vi "U8ToI32.vi"(4 "Index":u32, 7 "Input U8 Array":u8[](array[numeric])) -> (0 "Index+4":u32, 1 "Output I32":i32, 3 "Output U8 Array":u8[](array[numeric]))   [LabVIEW 2017]
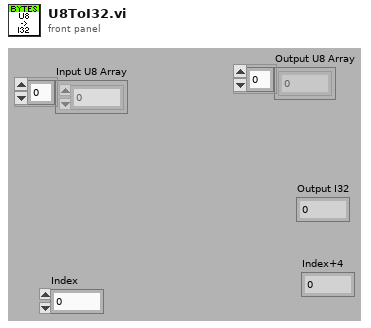
[diagram p1: front panel]
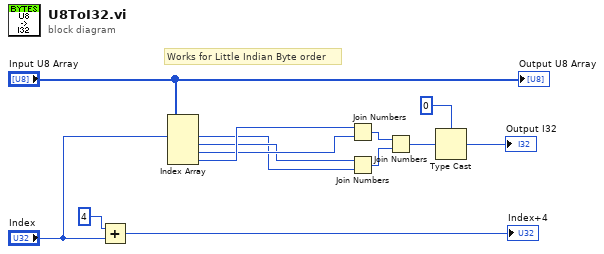
[diagram p0: block diagram]
diagram:
  # "Works for Little Indian Byte order"
  n1 = Add(x=4 ("count (1)"), y="Index") -> (x+y=→"Index+4":u32)
  n2 = Index Array(array="Input U8 Array", index #1="Index") -> (element #1=w6:u8, element #2=w7:u8, element #3=w8:u8, element #4=w9:u8)  [unwired: 3 in]
  n3 = Join Numbers(hi=w9, lo=w8) -> ((hi.lo)=w11:u16)
  n4 = Join Numbers(hi=w7, lo=w6) -> ((hi.lo)=w10:u16)
  n5 = Join Numbers(hi=w11, lo=w10) -> ((hi.lo)=w3:u32)
  n6 = Type Cast(type=0 ("count (1)"), x=w3) -> (*(type *) &x=→"Output I32":i32)
  "Output U8 Array" <- "Input U8 Array"
